vi "DSP_send_query.vi"(1 "CMD selection":T1(ring), 2 "GPIB address":string="0:12") -> (0 "Value":dbl)   [LabVIEW 2010]
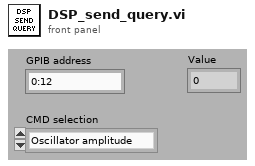
[diagram p1: front panel]
types:
  T1 = enum16{"Oscillator amplitude", "Oscillator frequency", "Sensitivity", "Time constant"}
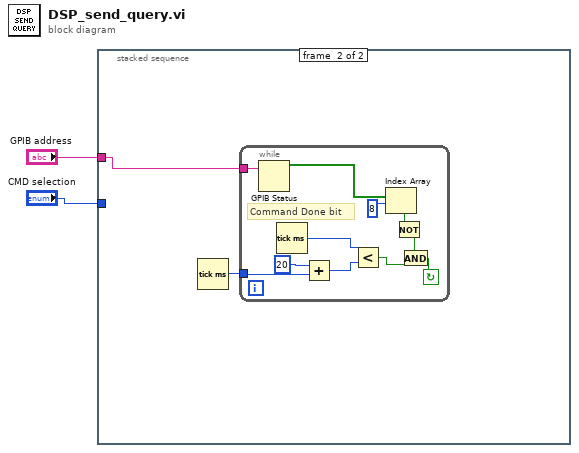
[diagram p0: block diagram]
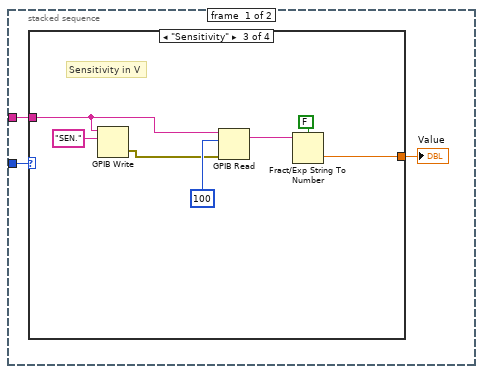
[diagram p2: hidden frame]
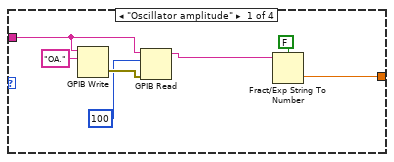
[diagram p3: hidden frame]
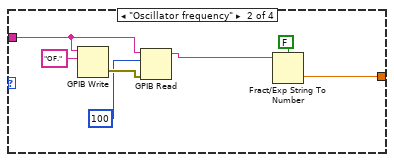
[diagram p4: hidden frame]
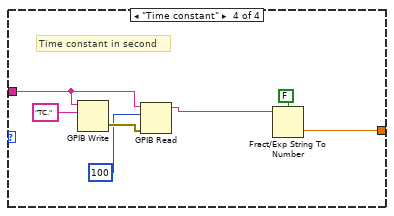
[diagram p5: hidden frame]
diagram:
  n1 = stacked-sequence {
    tunnel: "CMD selection" -> [w5 _]
    tunnel: "GPIB address" -> [w4 w34]
    frame #0 {
      n2 = case shown="\"Sensitivity\"" w5 {
        tunnel: w4 -> [w10 w17 w21 w31]
        tunnel: [w6 w13 w22 w27] -> w3
        frame "Oscillator amplitude" {
          n3 = GPIB Write(0:w10, 1:"OA.") -> (6:w11:errorcluster)  [unwired: 3 in, 1 out]
          n4 = GPIB Read(0:w10, 1:100, 3:w11) -> (5:w7:string)  [unwired: 2 in, 2 out]
          n5 = Fract/Exp String To Number(use system decimal point (T)=FALSE, string=w7) -> (number=w6:dbl)  [unwired: 2 in, 1 out]
        }
        frame "Oscillator frequency" {
          n6 = GPIB Write(0:w17, 1:"OF.") -> (6:w18:errorcluster)  [unwired: 3 in, 1 out]
          n7 = GPIB Read(0:w17, 1:100, 3:w18) -> (5:w14:string)  [unwired: 2 in, 2 out]
          n8 = Fract/Exp String To Number(use system decimal point (T)=FALSE, string=w14) -> (number=w13:dbl)  [unwired: 2 in, 1 out]
        }
        frame "Sensitivity" {
          # "Sensitivity in V"
          n9 = GPIB Write(0:w21, 1:"SEN.") -> (6:w20:errorcluster)  [unwired: 3 in, 1 out]
          n10 = GPIB Read(0:w21, 1:100, 3:w20) -> (5:w23:string)  [unwired: 2 in, 2 out]
          n11 = Fract/Exp String To Number(use system decimal point (T)=FALSE, string=w23) -> (number=w22:dbl)  [unwired: 2 in, 1 out]
        }
        frame "Time constant" {
          # "Time constant in second"
          n12 = GPIB Write(0:w31, 1:"TC.") -> (6:w32:errorcluster)  [unwired: 3 in, 1 out]
          n13 = GPIB Read(0:w31, 1:100, 3:w32) -> (5:w28:string)  [unwired: 2 in, 2 out]
          n14 = Fract/Exp String To Number(use system decimal point (T)=FALSE, string=w28) -> (number=w27:dbl)  [unwired: 2 in, 1 out]
        }
      }
      "Value" <- w3
    }
    frame #1 {
      n15 = Tick Count (ms)() -> (millisecond timer value=w35:u32)
      n16 = while {
        tunnel: w35 -> [w39]
        tunnel: w34 -> [w38]
        stop <- w41 continue-if-true
        # "Command Done bit"
        n17 = GPIB Status(0:w38) -> (2:w37:bool[])  [unwired: 1 in, 3 out]
        n18 = Tick Count (ms)() -> (millisecond timer value=w44:u32)
        n19 = Add(x=u32 20, y=w39) -> (x+y=w43:u32)
        n20 = Less?(x=w44, y=w43) -> (x < y?=w40:bool)
        n21 = Index Array(array=w37, index=8) -> (element=w45:bool)
        n22 = Not(x=w45) -> (.not. x?=w36:bool)
        n23 = And(x=w36, y=w40) -> (x .and. y?=w41:bool)
      }
    }
  }
